vi "Get Text From Clipboard.vi"() -> (0 "error out":errorcluster caption="에러 출력", 1 "Text From Clipboard":string)   [LabVIEW 2020]
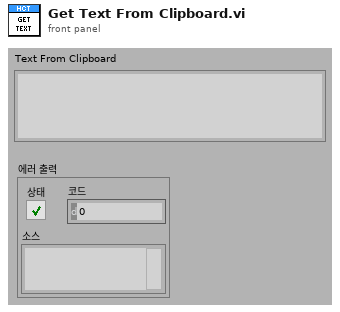
[diagram p1: front panel]
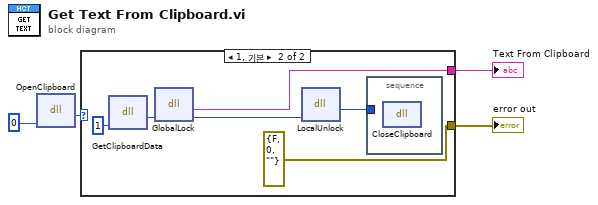
[diagram p0: block diagram]
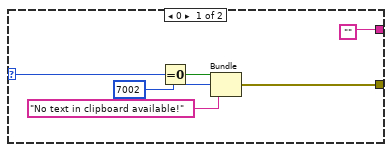
[diagram p2: hidden frame]
diagram:
  n1 = dll-call lib="user32" fn="OpenClipboard"("owner"=0) -> (w3:i32)  [unwired: 4 in, 2 out]
  n2 = case shown="1, 기본" w3 {
    selector: w3 -> [w6 _]
    tunnel: ["" w12] -> w2
    tunnel: [w7 cluster{bool, i32, "source":string} {FALSE, 0, "source"=""} ("Output Element")] -> w1
    frame 0 {
      n3 = Equal To 0?(x=w6) -> (x = 0?=w9:bool)
      n4 = Bundle(w9, 7002, "source"="No text in clipboard available!") -> (w7:cluster{bool, i32, "source":string})  [unwired: 1 in]
    }
    frame 1, Default {
      n5 = dll-call lib="user32" fn="GetClipboardData"("uFormat"=1 ("hGlobalMemory")) -> (w15:i32)  [unwired: 4 in, 2 out]
      n6 = dll-call lib="kernel32" fn="GlobalLock"("hGlobalMemory"=w15) -> (w12:string, "hGlobalMemory"=w14:i32)  [unwired: 3 in, 2 out]
      n7 = dll-call lib="kernel32" fn="LocalUnlock"("hGlobalMemory"=w14) -> (w13:i32)  [unwired: 4 in, 2 out]
      n8 = stacked-sequence {
        tunnel: w13 -> [_]
        frame #0 {
          n9 = dll-call lib="user32" fn="CloseClipboard"() -> ()  [unwired: 4 in, 2 out]
        }
      }
    }
  }
  "Text From Clipboard" <- w2
  "error out" <- w1
